vi "about.vi"(5 "parent":refnum<class "QWidget.lvclass">, 8 "Error In":errorcluster, 9 "text":string, 10 "title":string) -> (0 "Error Out":errorcluster)   [LabVIEW 2014, in "QMessageBox.lvclass"]
doc: "LabVIEW-specific documentation is not yet available. See <b>http://doc.qt.io/qt-5/QMessageBox.html#about</b>"
uses:
  QMessageBox.lvclass
  QWidget/QWidget.lvclass
  LQ Core/LQIdentity/LQIdentity.lvclass/LQIdentity.ctl
  LQ Core/LQ Core.lvlib
  LQ Core/LQIdentity/LQIdentity.lvclass
panel:
  # "Copyright (c) 2016 Sze Howe Koh\n\nThis Source Code Form is subject to the terms of the Mozilla Public\nLicense, v. 2.0. If a copy of the MPL was not distributed with this\nfile, You can obtain one at http://mozilla.org/MPL/2.0/."
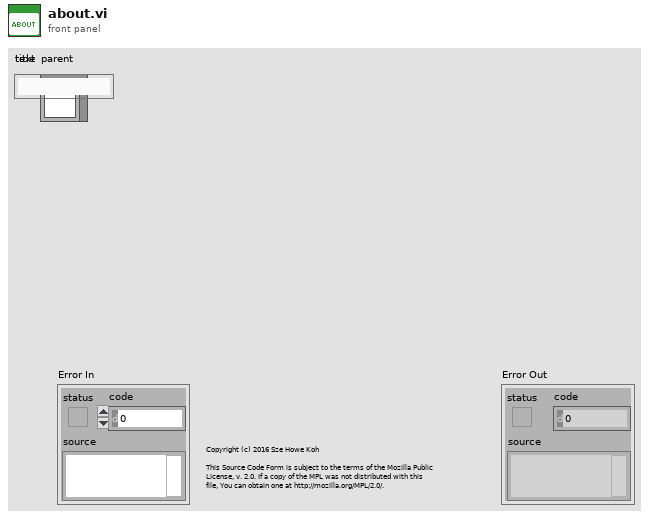
[diagram p1: front panel]
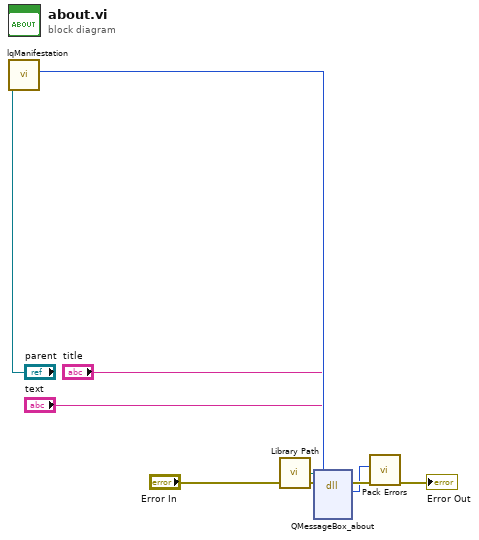
[diagram p0: block diagram]
diagram:
  n1 = call "lqManifestation.vi"("LQIdentity in"="parent") -> ("Manifestation"=w3:u64)  [unwired: 9 in, 1 out]
  n2 = call "Library Path.vi"() -> ("Library Path"=w9:path)
  n3 = dll-call lib="?" fn="QMessageBox_about"(path in=w9, error in="Error In", "parent"=w3, "title"="title", "text"="text") -> (error out=w7:errorcluster, w5:i32)  [unwired: 4 in, 1 out]
  n4 = call "Pack Errors.vi"("Error In"=w7, "Error Code"=w5) -> ("Error Out"=→"Error Out":errorcluster)  [unwired: 9 in]
